vi "Replace Template Literals.vi"(7 "Starting Offset (0)":u32, 8 "Error In":errorcluster, 11 "Path In":string) -> (0 "Error Out":errorcluster, 3 "Path Out":string)   [LabVIEW 2015, in "SystemLink runtime.lvclass"]
doc: "Resolve any template literals within path names. For example, when deployed on a target with the hostname \"cRIO-DCAF\", the input string \"${HOSTNAME}-TC0\" would output the string \"cRIO-DCAF-TC0\"."
uses:
  SystemLink runtime.lvclass
  <vilib>/regexp/Match Regular Expression.xnode
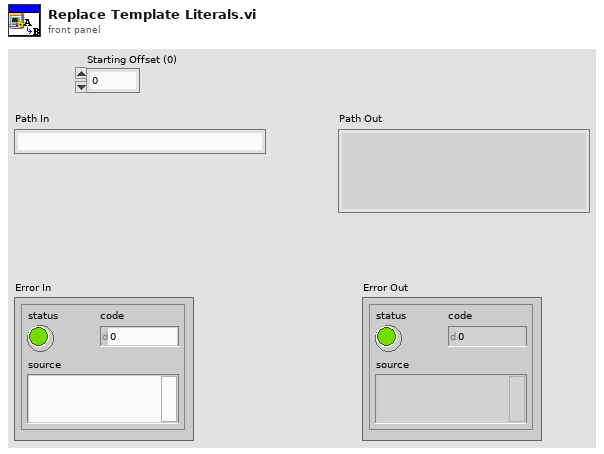
[diagram p1: front panel]
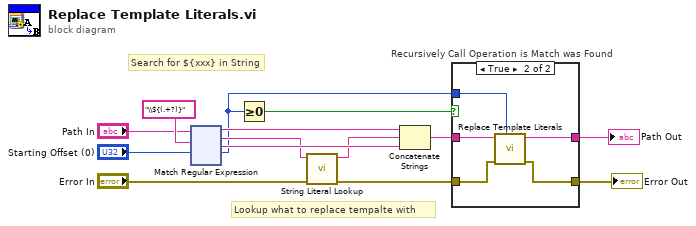
[diagram p0: block diagram]
diagram:
  # "Lookup what to replace tempalte with"
  # "Search for ${xxx} in String"
  n1 = xnode "Match Regular Expression"("input string"="Path In", "regular expression"="\\${(.+?)}", "offset (0)"="Starting Offset (0)") -> ("before match"=w12:string, "whole match"=w10:string, "after match"=w11:string, "offset past match"=w2:i32)  [unwired: 3 in, 1 out]
  n2 = Greater Or Equal To 0?(x=w2) -> (x >= 0?=w7:bool)
  n3 = call "String Literal Lookup.vi"("Error In"="Error In", "String Literal In"=w10) -> ("Error Out"=w6:errorcluster, "Resolved String"=w9:string)  [unwired: 8 in]
  n4 = Concatenate Strings(w12, w9, w11) -> (w5:string)
  n5 = case "Recursively Call Operation is Match was Found" shown="True" w7 {
    tunnel: w6 -> [w16 w20]
    tunnel: w5 -> [w15 w21]
    tunnel: [w16 w19] -> w4
    tunnel: [w15 w18] -> w3
    tunnel: w2 -> [_ w17]
    frame False {
    }
    frame True {
      n6 = call "Replace Template Literals.vi"("Starting Offset (0)"=w17, "Error In"=w20, "Path In"=w21) -> ("Error Out"=w19:errorcluster, "Path Out"=w18:string)  [unwired: 7 in]
    }
  }
  "Path Out" <- w3
  "Error Out" <- w4
